vi "PPCS_SIM_ENCODER_ALLOC.vi"() -> (3 "Encoder Index":T1)   [LabVIEW 2019]
uses:
  <vilib>/Rock Robotics/SystemInterfaces/Encoder/FPGA_EncoderIdx.ctl
  PPCS_SIM_SIM_Globals.vi
panel:
  # "PURPOSEFULLY NON-REENTRANT"
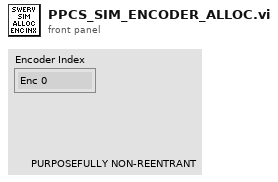
[diagram p1: front panel]
types:
  T1 = typedef "FPGA_EncoderIdx.ctl" = enum8{"Enc 0", "Enc 1", "Enc 2", "Enc 3", "Enc 4", "Enc 5", "Enc 6", "Enc 7", "Invalid"}
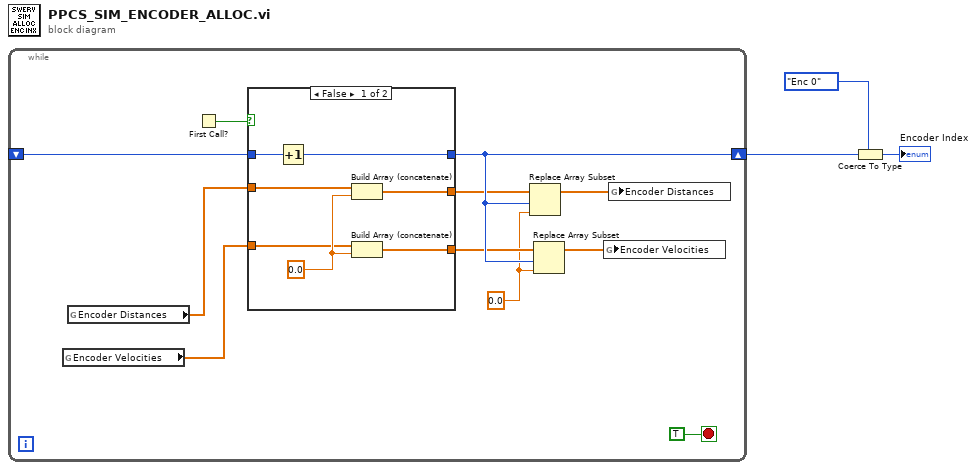
[diagram p0: block diagram]
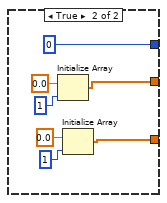
[diagram p2: hidden frame]
diagram:
  n1 = while {
    shift-right: [w11] -> w2
    shift-left: _ -> [w12]
    stop <- TRUE stop-if-true
    w8 = 0.0 ("new element/subarray")
    n2 = global read "PPCS_SIM_SIM_Globals.vi" "Encoder Velocities"() -> (w6:dbl[])
    n3 = global read "PPCS_SIM_SIM_Globals.vi" "Encoder Distances"() -> (w7:dbl[])
    n4 = First Call?() -> (First Call?: T/F=w13:bool)
    n5 = case shown="False" w13 {
      tunnel: [w20 0] -> w11
      tunnel: w12 -> [w21 _]
      tunnel: [w18 w23] -> w10
      tunnel: [w17 w22] -> w9
      tunnel: w7 -> [w16 _]
      tunnel: w6 -> [w15 _]
      frame False {
        w19 = 0.0 ("new element/subarray")
        n6 = Increment(x=w21) -> (x+1=w20:i32)
        n7 = Build Array (concatenate)(w16, w19) -> (w18:dbl[])
        n8 = Build Array (concatenate)(w15, w19) -> (w17:dbl[])
      }
      frame True {
        n9 = Initialize Array(0.0 ("element"), 1 ("dimension size")) -> (w23:dbl[])
        n10 = Initialize Array(0.0 ("element"), 1 ("dimension size")) -> (w22:dbl[])
      }
    }
    n11 = Replace Array Subset(array=w10, new element=w8, index=w11) -> (w5:dbl[])
    n12 = Replace Array Subset(array=w9, new element=w8, index=w11) -> (w4:dbl[])
    n13 = global write "PPCS_SIM_SIM_Globals.vi" "Encoder Velocities"(w4) -> ()
    n14 = global write "PPCS_SIM_SIM_Globals.vi" "Encoder Distances"(w5) -> ()
  }
  n15 = Coerce To Type(0:w2, 1:FPGA_EncoderIdx."Enc 0" ("EncoderIndex")) -> (2:→"Encoder Index":T1)
